vi "Constants.vi"() -> (0 "eo; Permitivity of Free Space":dbl=8.85418782e-12, 4 "c; Charge on e":dbl=1.6021766208e-19, 8 "k; Boltzmann Constant":dbl=1.38064852e-23, 12 "R=kN_a":dbl, 13 "F=eN_a":dbl, 14 "N_a; Avagadro no":dbl=1.38064852e-23)   [LabVIEW 2020]
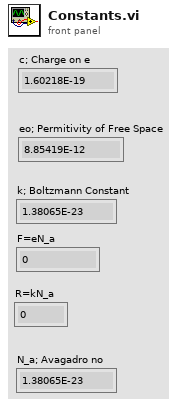
[diagram p1: front panel]
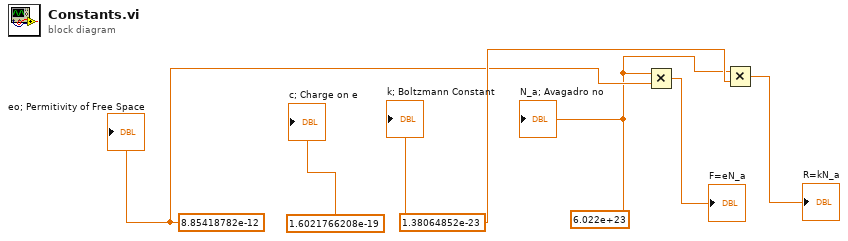
[diagram p0: block diagram]
diagram:
  w4 = 6.022e+23 ("x")
  w6 = 1.38064852e-23 ("x")
  w5 = 8.85418782e-12 ("y")
  n1 = Multiply(x=w4, y=w5) -> (x*y=→"F=eN_a":dbl)
  n2 = Multiply(x=w4, y=w6) -> (x*y=→"R=kN_a":dbl)
  "eo; Permitivity of Free Space" <- w5
  "k; Boltzmann Constant" <- w6
  "c; Charge on e" <- 1.6021766208e-19 ("x")
  "N_a; Avagadro no" <- w4
